vi "ScanRevised.vi"() -> ()   [LabVIEW 2023, in "HP4192A IA.lvclass"]
uses:
  HP4192A IA.lvclass
  <vilib>/Analysis/baseanly.llb/Mean (DBL).vi
  Global/GPIB Numbers.vi
  HP4192A Impedance Analyzer/HP4192 Impedance Analyzer.lvlib
  <vilib>/Analysis/NI_AALBase.lvlib
panel:
  out "dataTxt":string
  in  "Export\nPlot":bool
  in  "path":path
  out "error out":errorcluster
  in  "error in":errorcluster
  in  "Notes":string
  out "current numpoints":dbl
  in  "Take additional samples?":bool
  in  "number of samples in this range":i32=101
  in  "end freq for add'l sample":dbl[unit]=13000000.0
  in  "start freq for add'l samples":dbl[unit]=5.0
  in  "Total number of freq points":dbl=101.0
  in  "Final frequency":dbl[unit]=13000000.0
  in  "Initial frequency":dbl[unit]=5.0
  in  "Averaging?":bool
  out "Measurements vs. Frequency":cluster{"Y":dbl[], "Y":dbl[]}[](graph)=[{"Y"=[5.0, 5.0, 5.0, 5.0, 5.0], "Y"=[-246999.99999999997, -1063000.0, -361000.0, -401000.0, -539000.0]}]
  in  "Delay between\nsteps (ms)":u32=500
  in  "stop":bool
  out "Current Frequency":dbl[unit]
  in  "start":bool
  in  "L":bool
  in  "C":bool
  in  "R":bool
  in  "Z":bool
  # "Measure"
  # "Frequency range for additional samples"
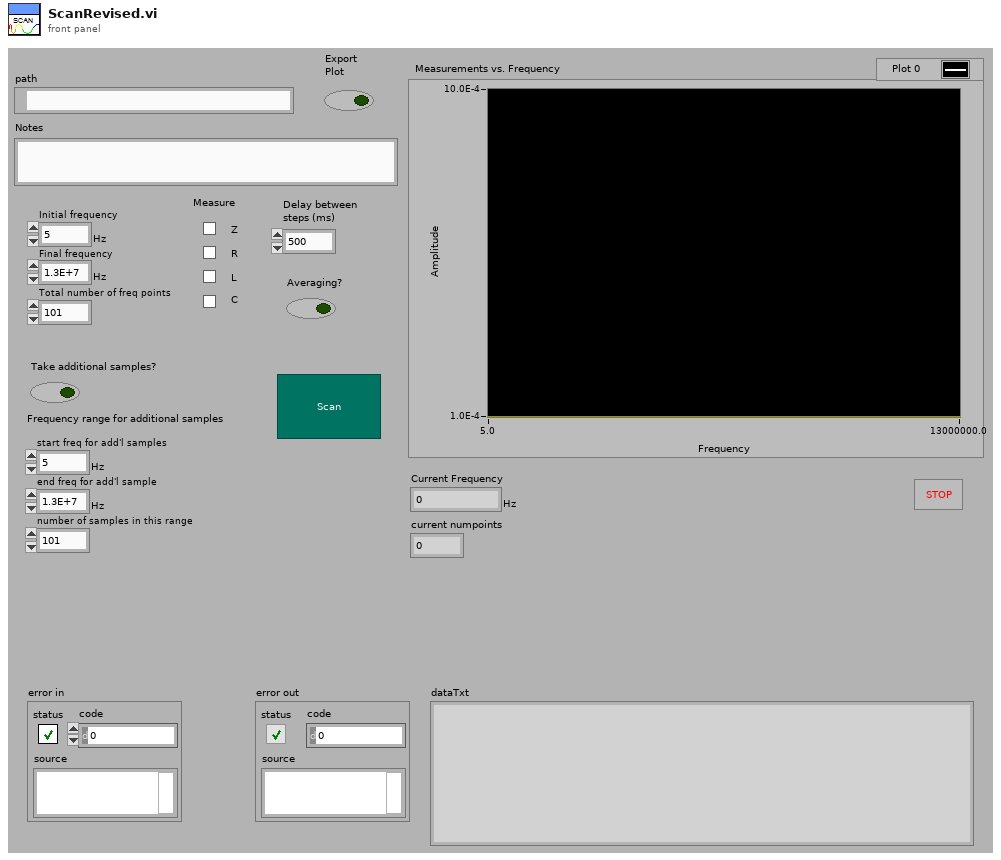
[diagram p1: front panel]
types:
  T1 = typedef "GPIB Type Def.ctl" = cluster{"Name":string, "bus":dbl, "GPIB":dbl, "GPIB as string":string, "byte":i32, "VISA Resource Name":refnum<visa-resource-name>}
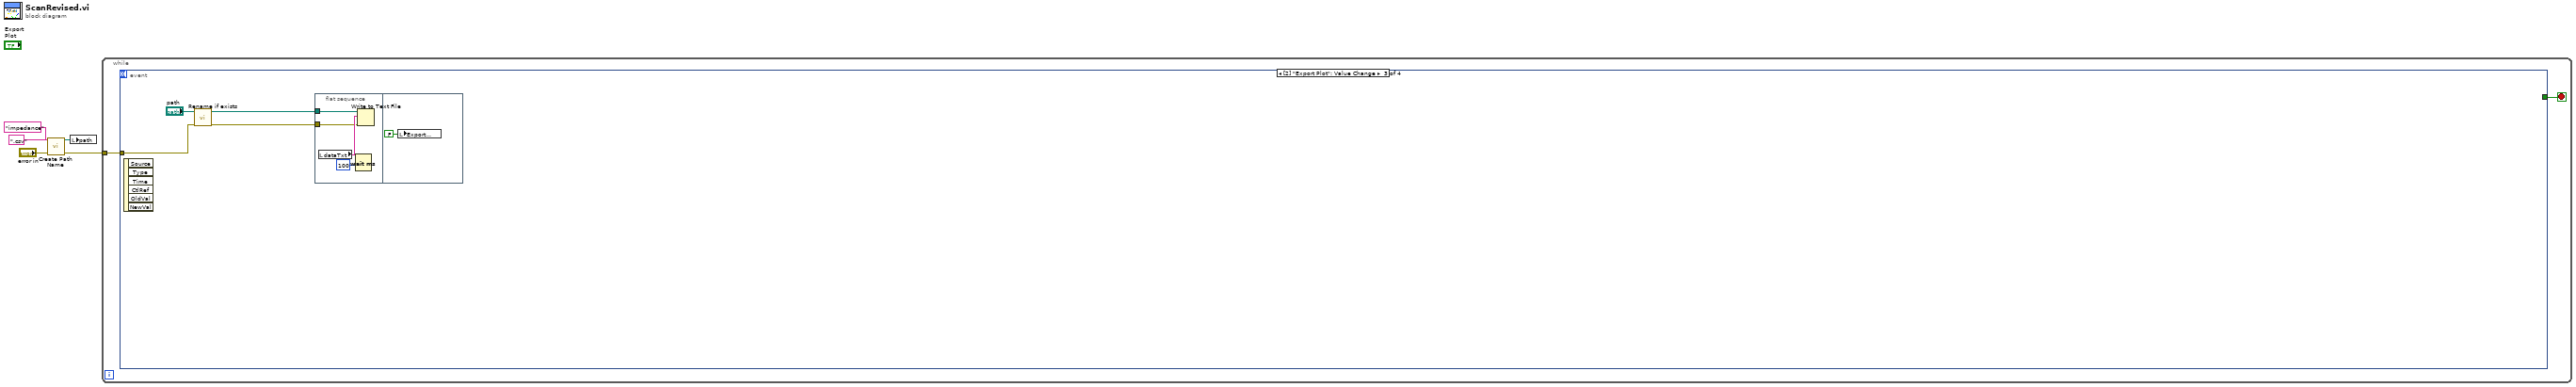
[diagram p0: block diagram]
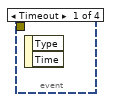
[diagram p2: hidden frame]
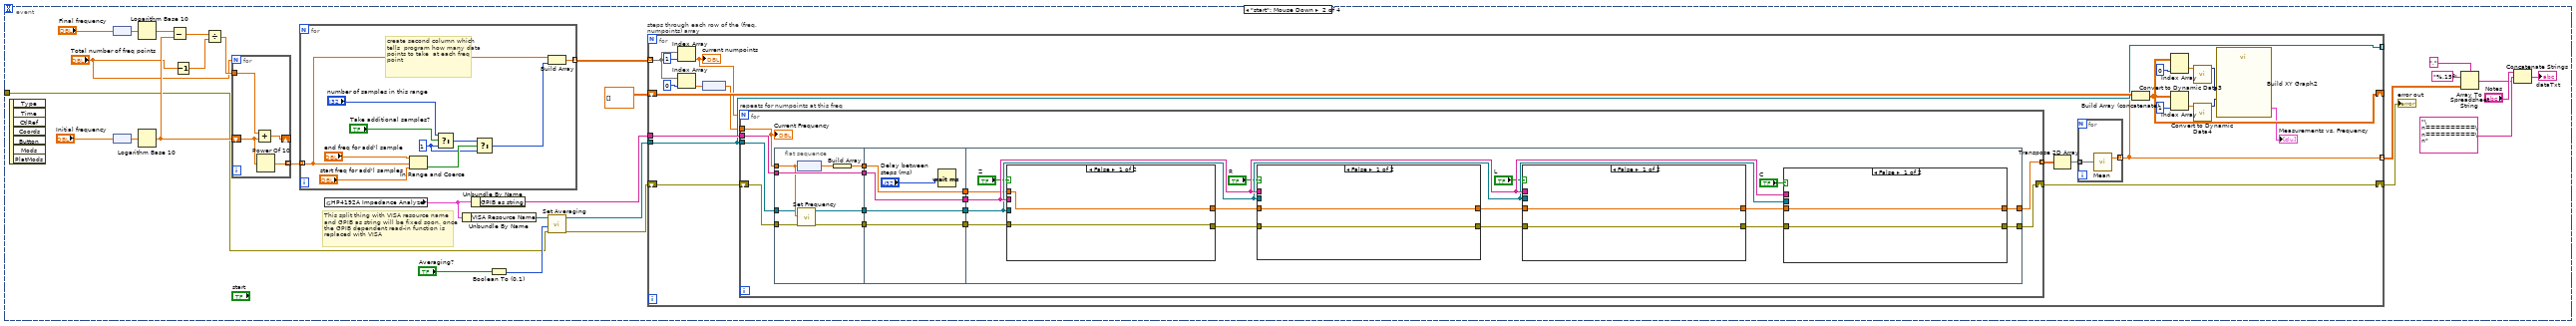
[diagram p3: hidden frame]
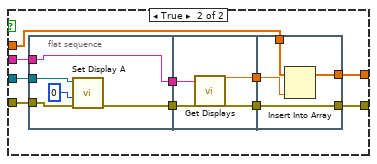
[diagram p4: hidden frame]
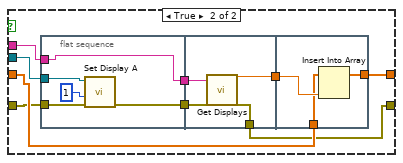
[diagram p5: hidden frame]
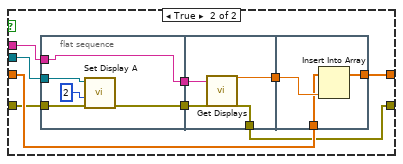
[diagram p6: hidden frame]
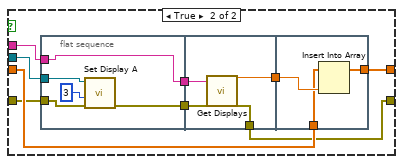
[diagram p7: hidden frame]
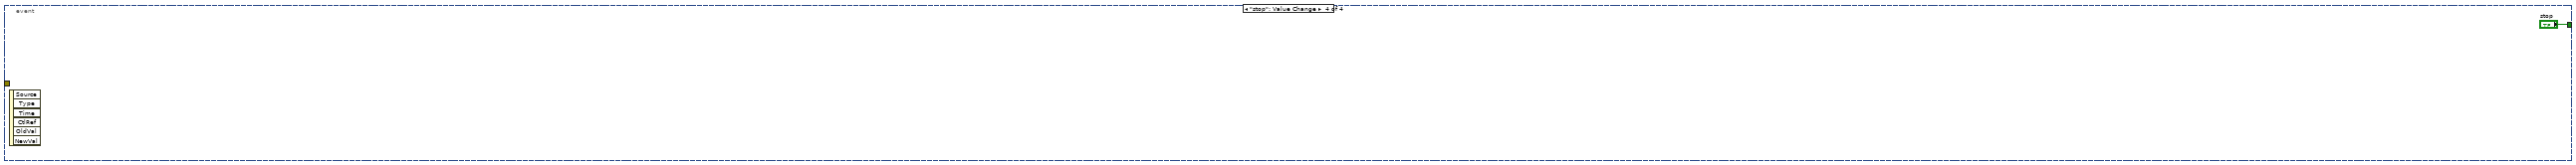
[diagram p8: hidden frame]
diagram:
  n1 = call "Create Path Name.vi"("error in"="error in", "String"=".csv", "filename"="impedance") -> ("error out"=w2:errorcluster, "path"=w4:path)  [unwired: 3 out]
  n2 = local write "path"(w4) -> ()
  n3 = while {
    tunnel: w2 -> [w6]
    stop <- w7 stop-if-true
    n4 = event shown="[2] \"Export Plot\": Value Change" {
      selector: _ -> [_ _ _ _]
      dyn-events: _ -> [_ _ _ _]
      timeout: _ -> [_ _ _ _]
      tunnel: [_ _ _ "stop"] -> w7
      tunnel: w6 -> [_ w8 w214 _]
      event Timeout {
        n5 = event-data() -> ()  [unwired: 1 in, 2 out]
      }
      event "start": Mouse Down {
        # "This split thing with VISA resource name  \nand GPIB as string will be fixed soon, once\nthe GPIB dependent read-in function is\nreplaced with VISA"
        n6 = event-data() -> ()  [unwired: 1 in, 7 out]
        n7 = node("Final frequency") -> (w23:dbl)
        n8 = node("Initial frequency") -> (w25:dbl)
        n9 = Logarithm Base 10(1:w23) -> (0:w30:dbl)
        n10 = Logarithm Base 10(1:w25) -> (0:w29:dbl)
        n11 = Subtract(x=w30, y=w29) -> (x-y=w35:dbl)
        n12 = Decrement(x="Total number of freq points") -> (x-1=w28:dbl)
        n13 = Divide(x=w35, y=w28) -> (x/y=w34:dbl)
        n14 = for {
          N: "Total number of freq points" -> [_]
          shift-right: [w211] -> _
          shift-left: w29 -> [w209]
          tunnel: w34 -> [w210]
          tunnel: [w208] -> w22 mode=indexing
          n15 = Add(x=w210, y=w209) -> (x+y=w211:dbl)
          n16 = Power Of 10(x=w209) -> (10^x=w208:dbl)
        }
        n17 = for {
          tunnel: w22 -> [w198] mode=indexing
          tunnel: [w199] -> w21 mode=indexing
          w202 = 1 ("f")
          # "create second column which tells  program how many data points to take  at each freq point"
          n18 = In Range and Coerce(upper limit="end freq for add'l sample", x=w198, lower limit="start freq for add'l samples") -> (In Range?=w205:bool)  [unwired: 1 out]
          n19 = Select(t="number of samples in this range", s="Take additional samples?", f=w202) -> (s? t:f=w201:i32)
          n20 = Select(t=w201, s=w205, f=w202) -> (s? t:f=w200:i32)
          n21 = Build Array(w198, w200) -> (w199:dbl[])
        }
        n22 = global read "GPIB Numbers.vi" "HP4192A Impedance Analyzer"() -> (w31:T1)
        n23 = Unbundle By Name(w31) -> ("VISA Resource Name"=w32:refnum<visa-resource-name>)
        n24 = Unbundle By Name(w31) -> ("GPIB as string"=w33:string)
        n25 = Boolean To (0,1)(Boolean="Averaging?") -> (0, 1=w18:i16)
        n26 = call "Set Averaging.vi"("error in (no error)"=w8, "Averaging"=w18, "VISA resource name"=w32) -> ("error out"=w10:errorcluster, "VISA resource name out"=w17:refnum<visa-resource-name>)  [unwired: 7 in]
        n27 = for "steps through each row of the (freq, numpoints) array" {
          tunnel: w21 -> [w45] mode=indexing
          tunnel: w33 -> [w58]
          tunnel: [w39] -> w36 mode=indexing
          shift-right: [w56] -> _
          shift-left: dbl[][] [] -> [w57]
          tunnel: [w55] -> _ mode=indexing
          tunnel: w17 -> [w55]
          shift-right: [w37] -> w9
          shift-left: w10 -> [w38]
          n28 = Index Array(array=w45, index=1) -> (element=w47:dbl)
          "current numpoints" <- w47
          n29 = Index Array(array=w45, index=0) -> (element=w43:dbl)
          n30 = node(w43) -> (w42:dbl[unit])
          n31 = for "repeats for numpoints at this freq" {
            N: w47 -> [_]
            tunnel: w58 -> [w68]
            tunnel: w42 -> [w67]
            tunnel: [w66] -> w41 mode=indexing
            tunnel: w55 -> [w65]
            shift-right: [w61] -> w37
            shift-left: w38 -> [w64]
            n32 = flat-sequence {
              tunnel: w68 -> [w80]
              tunnel: [w80] -> w74
              tunnel: w67 -> [w79]
              tunnel: [w82] -> w73
              tunnel: w65 -> [w78]
              tunnel: [w77] -> w72
              tunnel: w64 -> [w76]
              tunnel: [w75] -> w62
              tunnel: w74 -> [w86]
              tunnel: [w86] -> w71
              tunnel: w73 -> [w85]
              tunnel: [w85] -> w70
              tunnel: [w84] -> w69
              tunnel: w72 -> [w84]
              tunnel: [w83] -> w63
              tunnel: w62 -> [w83]
              tunnel: [w101] -> w66
              tunnel: [w97] -> w61
              tunnel: w63 -> [w88]
              tunnel: w69 -> [w99]
              tunnel: w70 -> [w90]
              tunnel: w71 -> [w103]
              frame #0 {
                n33 = node(w79) -> (w81:dbl)
                n34 = call "Set Frequency.vi"("error in (no error)"=w76, "test signal freq"=w79, "VISA resource name"=w78) -> ("error out"=w75:errorcluster, "VISA resource name out"=w77:refnum<visa-resource-name>)  [unwired: 7 in]
                n35 = Build Array(w81) -> (w82:dbl[])
              }
              frame #1 {
                n36 = Wait (ms)(milliseconds to wait="Delay between\nsteps (ms)") -> ()  [unwired: 1 out]
              }
              frame #2 {
                n37 = case shown="False" "Z" {
                  tunnel: w90 -> [w105 w113]
                  tunnel: w103 -> [_ w115]
                  tunnel: [w105 w112] -> w93
                  tunnel: w99 -> [_ w111]
                  tunnel: w88 -> [w104 w109]
                  tunnel: [w104 w106] -> w91
                  frame False {
                  }
                  frame True {
                    n38 = flat-sequence {
                      tunnel: w111 -> [w119]
                      tunnel: w115 -> [w120]
                      tunnel: [w120] -> w110
                      tunnel: w109 -> [w117]
                      tunnel: [w116] -> w108
                      tunnel: [w123] -> w114
                      tunnel: w110 -> [w124]
                      tunnel: w108 -> [w122]
                      tunnel: [w121] -> w107
                      tunnel: w114 -> [w127]
                      tunnel: w113 -> [w128]
                      tunnel: [w126] -> w112
                      tunnel: [w125] -> w106
                      tunnel: w107 -> [w125]
                      frame #0 {
                        n39 = call "Set Display A.vi"("error in (no error)"=w117, "function A (z/y:0)"=i16 0, "VISA resource name"=w119) -> ("error out 2"=w116:errorcluster)  [unwired: 8 in]
                      }
                      frame #1 {
                        n40 = call "Get Displays.vi"("GPIB addess"=w124, "error in (no error)"=w122) -> ("display A"=w123:dbl, "error out"=w121:errorcluster)  [unwired: 17 in, 7 out]
                      }
                      frame #2 {
                        n41 = Insert Into Array(array=w128, new element=w127) -> (w126:dbl[])  [unwired: 1 in]
                      }
                    }
                  }
                }
                n42 = case shown="False" "R" {
                  tunnel: w103 -> [_ w138]
                  tunnel: w93 -> [w130 w137]
                  tunnel: [w130 w136] -> w96
                  tunnel: w99 -> [_ w134]
                  tunnel: w91 -> [w129 w133]
                  tunnel: [w129 w131] -> w94
                  frame False {
                  }
                  frame True {
                    n43 = flat-sequence {
                      tunnel: w138 -> [w144]
                      tunnel: [w144] -> w135
                      tunnel: w134 -> [w142]
                      tunnel: w133 -> [w141]
                      tunnel: [w140] -> w132
                      tunnel: [w148] -> w139
                      tunnel: w135 -> [w147]
                      tunnel: w132 -> [w146]
                      tunnel: [w145] -> w131
                      tunnel: w139 -> [w151]
                      tunnel: w137 -> [w150]
                      tunnel: [w149] -> w136
                      frame #0 {
                        n44 = call "Set Display A.vi"("error in (no error)"=w141, "function A (z/y:0)"=i16 1, "VISA resource name"=w142) -> ("error out 2"=w140:errorcluster)  [unwired: 8 in]
                      }
                      frame #1 {
                        n45 = call "Get Displays.vi"("GPIB addess"=w147, "error in (no error)"=w146) -> ("display A"=w148:dbl, "error out"=w145:errorcluster)  [unwired: 17 in, 7 out]
                      }
                      frame #2 {
                        n46 = Insert Into Array(array=w150, new element=w151) -> (w149:dbl[])  [unwired: 1 in]
                      }
                    }
                  }
                }
                n47 = case shown="False" "L" {
                  tunnel: [w153 w161] -> w102
                  tunnel: w96 -> [w153 w160]
                  tunnel: w103 -> [_ w159]
                  tunnel: w99 -> [_ w157]
                  tunnel: w94 -> [w152 w156]
                  tunnel: [w152 w154] -> w98
                  frame False {
                  }
                  frame True {
                    n48 = flat-sequence {
                      tunnel: w159 -> [w167]
                      tunnel: [w167] -> w158
                      tunnel: w157 -> [w165]
                      tunnel: w156 -> [w164]
                      tunnel: [w163] -> w155
                      tunnel: [w171] -> w162
                      tunnel: w158 -> [w170]
                      tunnel: w155 -> [w169]
                      tunnel: [w168] -> w154
                      tunnel: w162 -> [w174]
                      tunnel: [w173] -> w161
                      tunnel: w160 -> [w172]
                      frame #0 {
                        n49 = call "Set Display A.vi"("error in (no error)"=w164, "function A (z/y:0)"=i16 2, "VISA resource name"=w165) -> ("error out 2"=w163:errorcluster)  [unwired: 8 in]
                      }
                      frame #1 {
                        n50 = call "Get Displays.vi"("GPIB addess"=w170, "error in (no error)"=w169) -> ("display A"=w171:dbl, "error out"=w168:errorcluster)  [unwired: 17 in, 7 out]
                      }
                      frame #2 {
                        n51 = Insert Into Array(array=w172, new element=w174) -> (w173:dbl[])  [unwired: 1 in]
                      }
                    }
                  }
                }
                n52 = case shown="False" "C" {
                  tunnel: [w176 w184] -> w101
                  tunnel: w103 -> [_ w183]
                  tunnel: w102 -> [w176 w182]
                  tunnel: w99 -> [_ w180]
                  tunnel: w98 -> [w175 w179]
                  tunnel: [w175 w177] -> w97
                  frame False {
                  }
                  frame True {
                    n53 = flat-sequence {
                      tunnel: w183 -> [w190]
                      tunnel: [w190] -> w181
                      tunnel: w180 -> [w188]
                      tunnel: w179 -> [w187]
                      tunnel: [w186] -> w178
                      tunnel: [w194] -> w185
                      tunnel: w181 -> [w193]
                      tunnel: w178 -> [w192]
                      tunnel: [w191] -> w177
                      tunnel: w185 -> [w197]
                      tunnel: [w196] -> w184
                      tunnel: w182 -> [w195]
                      frame #0 {
                        n54 = call "Set Display A.vi"("error in (no error)"=w187, "function A (z/y:0)"=i16 3, "VISA resource name"=w188) -> ("error out 2"=w186:errorcluster)  [unwired: 8 in]
                      }
                      frame #1 {
                        n55 = call "Get Displays.vi"("GPIB addess"=w193, "error in (no error)"=w192) -> ("display A"=w194:dbl, "error out"=w191:errorcluster)  [unwired: 17 in, 7 out]
                      }
                      frame #2 {
                        n56 = Insert Into Array(array=w195, new element=w197) -> (w196:dbl[])  [unwired: 1 in]
                      }
                    }
                  }
                }
              }
            }
            "Current Frequency" <- w67
          }
          n57 = Transpose 2D Array(2D array=w41) -> (transposed array=w40:dbl[][])
          n58 = for {
            tunnel: w40 -> [w60] mode=indexing
            tunnel: [w59] -> w39 mode=indexing
            n59 = call-poly <vilib>:"Mean.vi"("X"=w60) -> ("mean"=w59:dbl)  [unwired: 1 out]
          }
          n60 = Build Array (concatenate)(w57, w39) -> (w56:dbl[][])
          n61 = Index Array(array=w56, index (col)=0) -> (element=w49:dbl[])  [unwired: 1 in]
          n62 = Index Array(array=w56, index (col)=1) -> (element=w48:dbl[])  [unwired: 1 in]
          n63 = call "Convert to Dynamic Data3"("Array"=w49) -> ("Dynamic Data Type"=w50:dynamicdata)  [unwired: 3 in]
          n64 = call "Convert to Dynamic Data4"("Array"=w48) -> ("Dynamic Data Type"=w51:dynamicdata)  [unwired: 3 in]
          n65 = call "Build XY Graph2"("Y Input"=w51, "X Input"=w50) -> ("XY Graph"=→"Measurements vs. Frequency":cluster{"Y":dbl[], "Y":dbl[]}[])  [unwired: 8 in, 1 out]
        }
        "error out" <- w9
        n66 = Array To Spreadsheet String(delimiter (Tab)=",", array=w36, 3:"%.15f") -> (spreadsheet string=w13:string)
        n67 = Concatenate Strings("Notes", "\n==========\n==========\n" ("string"), w13) -> (→"dataTxt":string)
      }
      event "Export\nPlot": Value Change {
        n68 = event-data() -> ()  [unwired: 1 in, 6 out]
        n69 = call "Rename if exists.vi"("error in"=w214, "File Path"="path") -> ("error out"=w212:errorcluster, "New path"=w213:path)  [unwired: 1 in, 7 out]
        n70 = flat-sequence {
          tunnel: w213 -> [w218]
          tunnel: w212 -> [w217]
          frame #0 {
            n71 = local read "dataTxt"() -> (w219:string)
            n72 = Wait (ms)(milliseconds to wait=u32 100) -> ()  [unwired: 1 out]
            n73 = Write to Text File(file (use dialog)=w218, text=w219, error in=w217) -> ()  [unwired: 1 in, 3 out]
          }
          frame #1 {
            n74 = local write "Export\nPlot"(FALSE ("Export\nPlot")) -> ()
          }
        }
      }
      event "stop": Value Change {
        n75 = event-data() -> ()  [unwired: 1 in, 6 out]
      }
    }
  }
